vi "RT_rotation (SubVI).vi"(4 "W(i) (rad/s) in":dbl[](array[numeric]), 6 "q(i) in":dbl[](array[numeric]), 8 "W_b(i)":dbl[](array[numeric]), 9 "ang_acc":dbl[](array[numeric]), 10 "dt":dbl, 11 "dt*0.5":dbl) -> (2 "W(i+1)":dbl[](array[numeric]), 3 "q(i+1)":dbl[](array[numeric]))   [LabVIEW 2017]
uses:
  <vilib>/Analysis/_algsub.llb/Vector Norm Type.ctl
  <vilib>/Analysis/_algsub.llb/Real Vector Norm.vi
  <vilib>/Analysis/baseanly.llb/Real A x B.vi
  <vilib>/Analysis/Matrix/Numeric/Conversions/Array To Matrix - RA2.vi
  <vilib>/Analysis/Matrix/Numeric/Conversions/Array To Matrix - RA.vi
  <vilib>/Analysis/Matrix/Numeric/Conversions/Matrix To Array - RM.vi
  <vilib>/Analysis/Matrix/NI_Matrix.lvlib
  <vilib>/Analysis/NI_AALBase.lvlib
  <vilib>/Analysis/NI_AALPro.lvlib
panel:
  out "Exp_Omega_k_T":dbl[][](array[numeric])
  out "S":dbl[][](array[numeric])
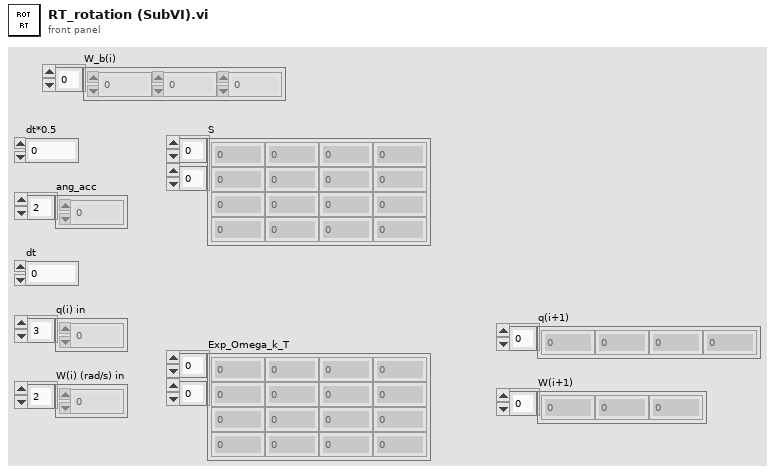
[diagram p1: front panel]
types:
  T1 = typedef "NI_AALPro.lvlib/Vector Norm Type.ctl" = u16
  T2 = typedef "NI_Matrix.lvlib/RealMatrix.ctl" = dbl[][]
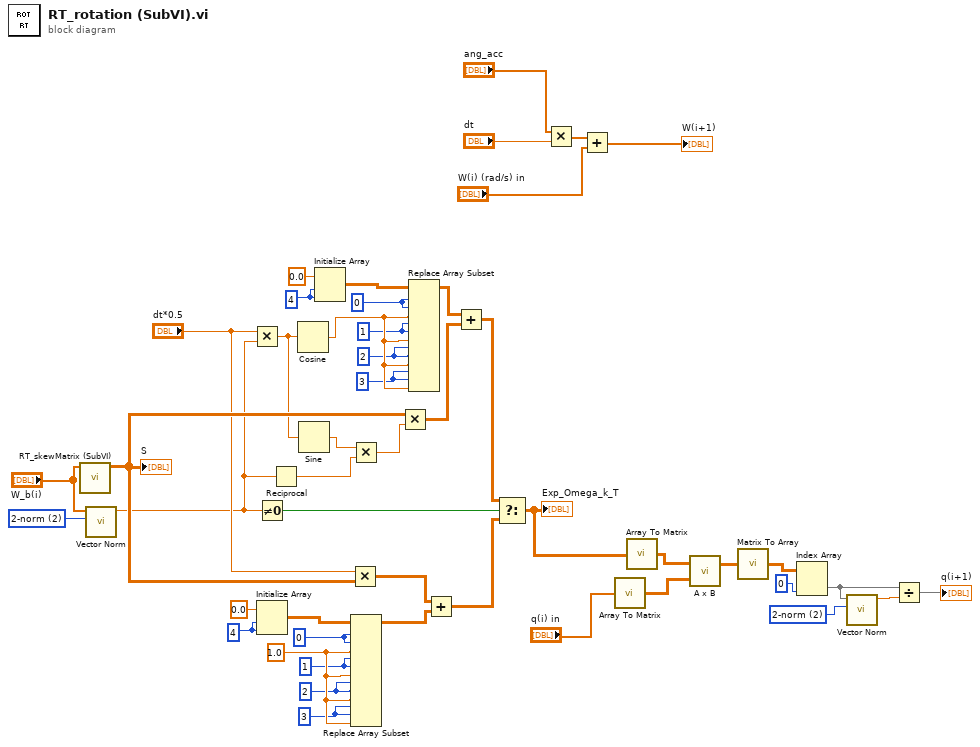
[diagram p0: block diagram]
diagram:
  w41 = T1 2 items=["1-norm"=1, "2-norm"=2, "Inf-norm"=3, "-Inf-norm"=4, "User Defined"=5] ("norm type")
  w29 = 1.0 ("new element/subarray")
  w24 = 3 ("disabled index (row)")
  w23 = 2 ("disabled index (row)")
  w22 = 1 ("disabled index (row)")
  w25 = 0 ("disabled index (row)")
  w28 = 4 ("dimension size")
  w17 = 3 ("disabled index (row)")
  w18 = 2 ("disabled index (row)")
  w19 = 1 ("disabled index (row)")
  w16 = 0 ("disabled index (row)")
  w6 = 4 ("dimension size")
  w3 = T1 2 items=["1-norm"=1, "2-norm"=2, "Inf-norm"=3, "-Inf-norm"=4, "User Defined"=5] ("norm type")
  n1 = call "RT_skewMatrix (SubVI).vi"("vector"="W_b(i)") -> ("skew matrix"=w31:dbl[][])  [unwired: 10 in]
  "S" <- w31
  n2 = call-poly <vilib>:"Vector Norm.vi"("norm type"=w3, "Input Vector"="W_b(i)") -> ("norm"=w9:dbl)  [unwired: 8 in, 1 out]
  n3 = Multiply(x="dt*0.5", y=w9) -> (x*y=w8:dbl)
  n4 = Not Equal To 0?(x=w9) -> (x != 0?=w5:bool)
  n5 = Initialize Array(0.0 ("element"), w28, w28) -> (w26:dbl[][])
  n6 = Reciprocal(x=w9) -> (1/x=w11:dbl)
  n7 = Cosine(x=w8) -> (cos(x)=w20:dbl)
  n8 = Sine(x=w8) -> (sin(x)=w10:dbl)
  n9 = Initialize Array(0.0 ("element"), w6, w6) -> (w14:dbl[][])
  n10 = Multiply(x="dt*0.5", y=w31) -> (x*y=w32:dbl[][])
  n11 = Multiply(x=w10, y=w11) -> (x*y=w12:dbl)
  n12 = Replace Array Subset(array=w26, new element #1=w29, index (row) #1=w25, index (col) #1=w25, new element #2=w29, index (row) #2=w22, index (col) #2=w22, new element #3=w29, index (row) #3=w23, index (col) #3=w23, new element #4=w29, index (row) #4=w24, index (col) #4=w24) -> (w33:dbl[][])
  n13 = Multiply(x=w31, y=w12) -> (x*y=w13:dbl[][])
  n14 = Replace Array Subset(array=w14, new element #1=w20, index (row) #1=w16, index (col) #1=w16, new element #2=w20, index (row) #2=w19, index (col) #2=w19, new element #3=w20, index (row) #3=w18, index (col) #3=w18, new element #4=w20, index (row) #4=w17, index (col) #4=w17) -> (w15:dbl[][])
  n15 = Add ("Add.vi")(x=w32, y=w33) -> (x+y=w34:dbl[][])
  n16 = Add ("Add.vi")(x=w15, y=w13) -> (x+y=w21:dbl[][])
  n17 = Select(t=w21, s=w5, f=w34) -> (s? t:f=w40:dbl[][])
  "Exp_Omega_k_T" <- w40
  n18 = Multiply(x="ang_acc", y="dt") -> (x*y=w47:dbl[])
  n19 = Add ("Add.vi")(x=w47, y="W(i) (rad/s) in") -> (x+y=→"W(i+1)":dbl[])
  n20 = call-poly <vilib>:"Array To Matrix.vi"("Real 1D Array"="q(i) in") -> ("Real Matrix (Column Vector)"=w38:T2)
  n21 = call-poly <vilib>:"Array To Matrix.vi"("Real 2D Array"=w40) -> ("Real Matrix"=w39:T2)
  n22 = call-poly <vilib>:"A x B.vi"("B"=w38, "A"=w39) -> ("A x B"=w36:T2)  [unwired: 1 out]
  n23 = call-poly <vilib>:"Matrix To Array.vi"("Real Matrix"=w36) -> ("Real 2D Array"=w37:dbl[][])
  n24 = Index Array(array=w37, index (col)=0 ("index (row)")) -> (element=w43:dbl[])  [unwired: 1 in]
  n25 = call-poly <vilib>:"Vector Norm.vi"("norm type"=w41, "Input Vector"=w43) -> ("norm"=w42:dbl)  [unwired: 8 in, 1 out]
  n26 = Divide(x=w43, y=w42) -> (x/y=→"q(i+1)":dbl[])
